vi "F2tauScale.vi"(8 "F2 channel":u8, 9 "Palette tau":T3(ring), 10 "Palette F2":T3(ring), 11 "Enum":T1(ring)) -> (0 "error out":errorcluster, 2 "tauscale":T2, 3 "F2-scale":T2, 4 "title tau":string, 5 "title F2":string)   [LabVIEW 2009]
uses:
  <vilib>/vision/Image Controls.llb/IMAQ Image.ctl
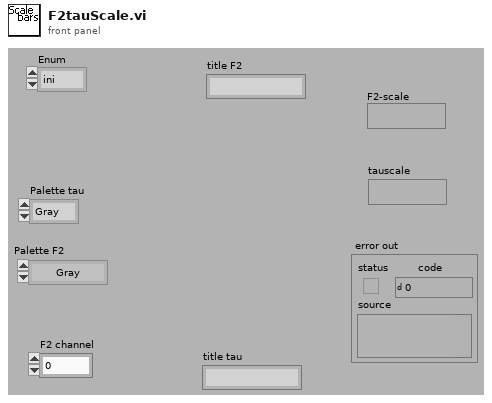
[diagram p1: front panel]
types:
  T1 = enum16{"ini", "get", "change", "export", "draw", "dump", "kill", "colorpal"}
  T2 = typedef "IMAQ Image.ctl" = refnum<image>
  T3 = enum32{"Gray", "Binary", "Gradient", "Rainbow", "Temperature"}
  T4 = typedef "Settings.ctl" = cluster{"threshold":cluster{"max":u32, "min":u32}, "RGB or false color":bool, "16bit":bool, "log/lin axis":u16, "spotsize button":bool, "Pixelsize":u16, "autoscale x":bool, "autoscale y":bool, "correlation":bool, "ADC-Resolution":i32, "F2-lifetime":cluster{"display tau":bool, "display F2":bool, "Palette Number lifetime":enum32{"Gray", "Binary", "Gradient", "Rainbow", "Temperature"}, "Palette Number F2":enum32{"Gray", "Binary", "Gradient", "Rainbow", "Temperature"}, "max tau-Value":dbl, "min tau-Value":dbl, "max F2-Value":dbl, "min F2-Value":dbl}, "TAC-Window 1":u16, "TAC-Window 2":u16, "false color palette":cluster{"1":u32, "2":u32, "3":u32, "4":u32, "5":u32, "6":u32, "7":u32, "8":u32, "8 2":u32, "8 3":u32, "8 4":u32, "8 5":u32}}
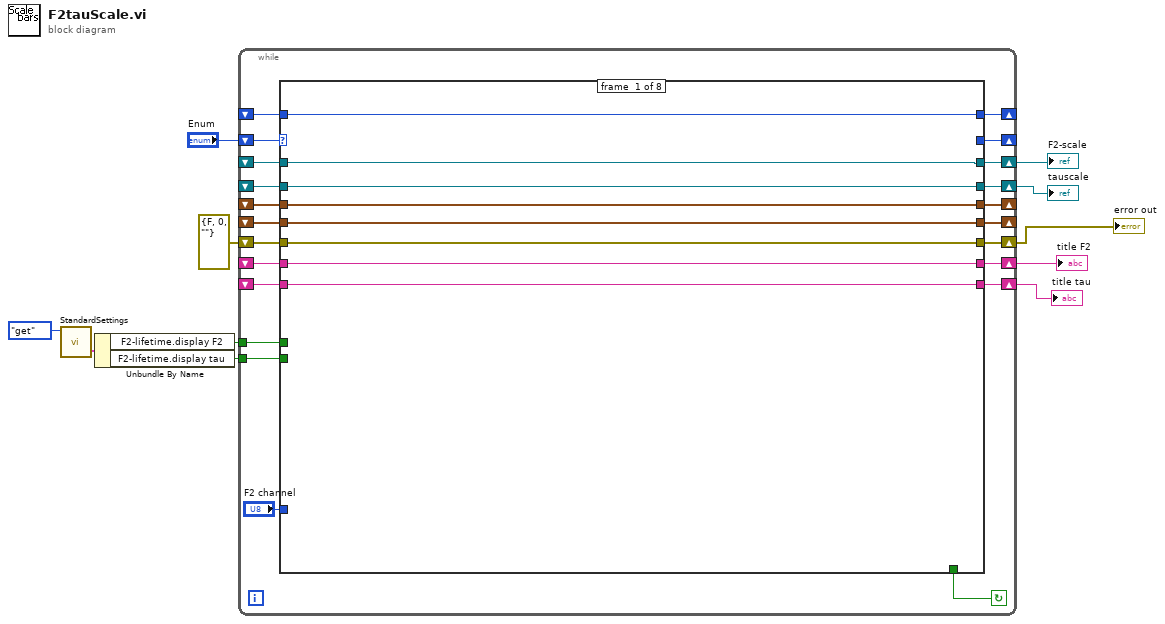
[diagram p0: block diagram]
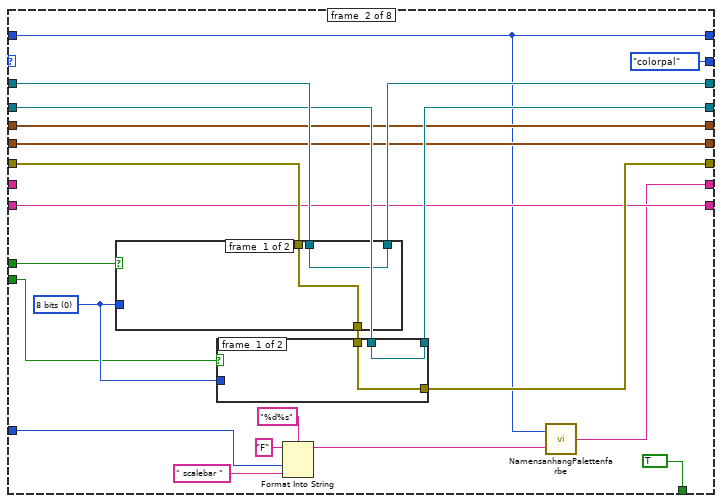
[diagram p2: hidden frame]
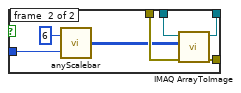
[diagram p3: hidden frame]
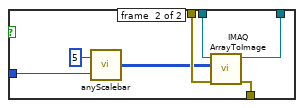
[diagram p4: hidden frame]
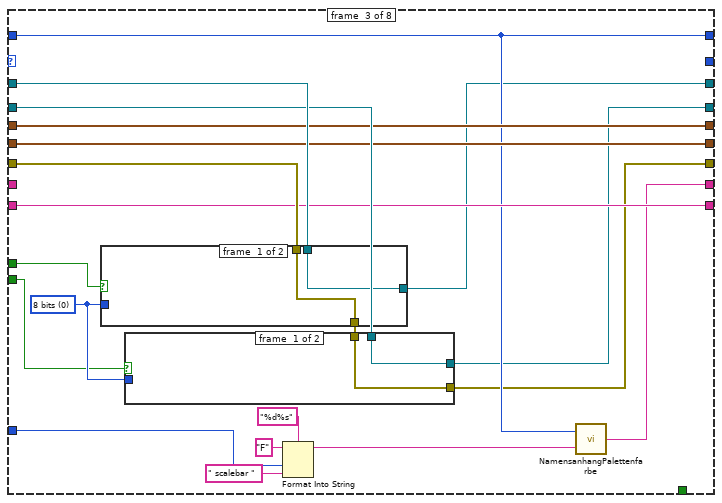
[diagram p5: hidden frame]
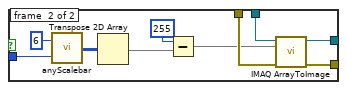
[diagram p6: hidden frame]
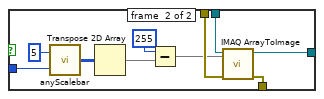
[diagram p7: hidden frame]
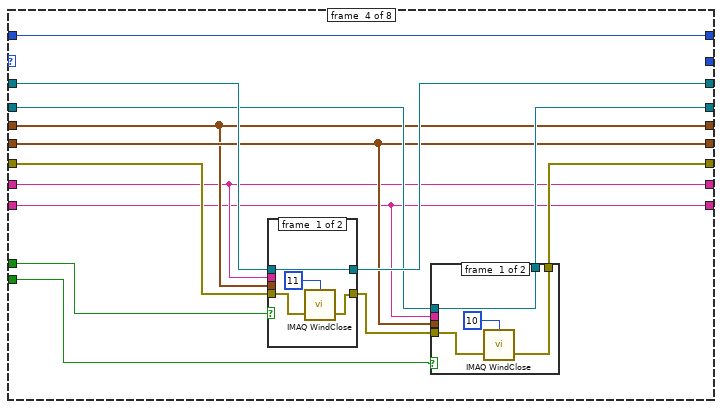
[diagram p8: hidden frame]
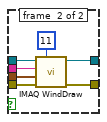
[diagram p9: hidden frame]
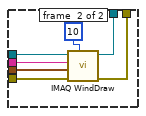
[diagram p10: hidden frame]
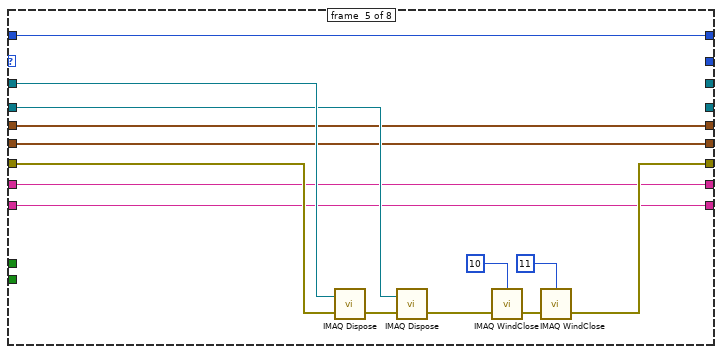
[diagram p11: hidden frame]
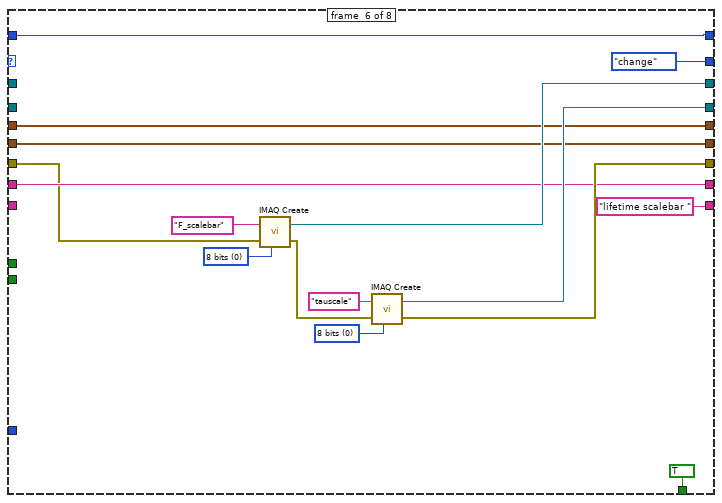
[diagram p12: hidden frame]
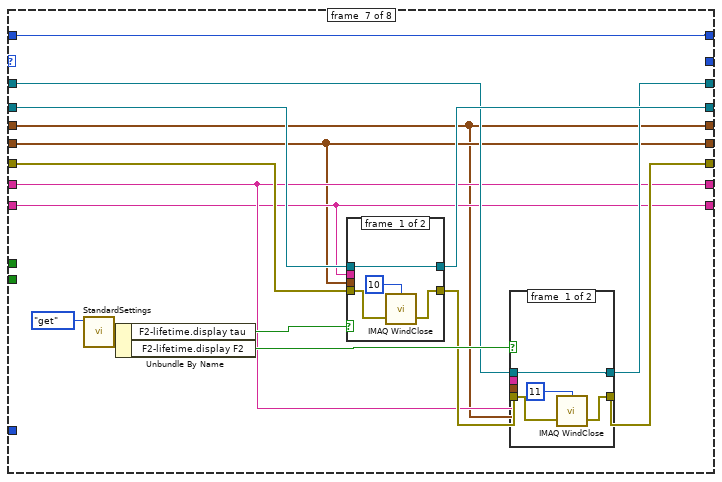
[diagram p13: hidden frame]
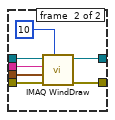
[diagram p14: hidden frame]
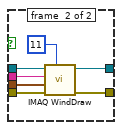
[diagram p15: hidden frame]
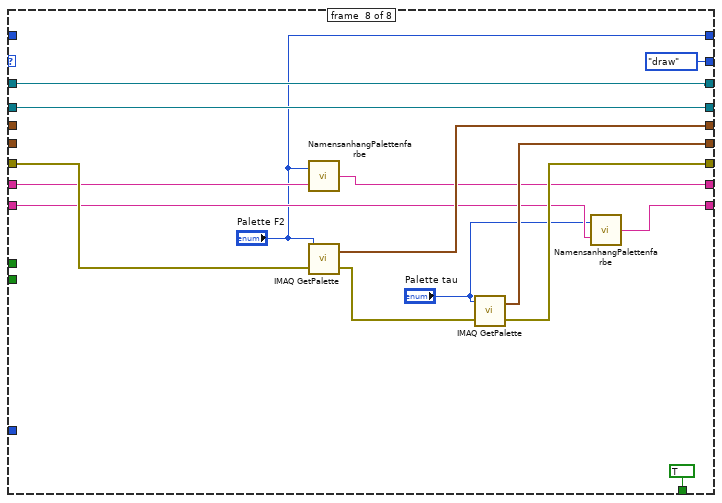
[diagram p16: hidden frame]
diagram:
  n1 = call "StandardSettings.vi"("Enum"=enum16{"Load", "get", "Save", "set"}."get") -> ("StandardSettings"=w3:T4)  [unwired: 4 in]
  n2 = Unbundle By Name(w3) -> ("F2-lifetime.display F2"=w2:bool, "F2-lifetime.display tau"=w1:bool)
  n3 = while {
    shift-right: [w32] -> _
    shift-left: "Enum" -> [w33]
    shift-right: [w31] -> w10
    shift-left: _ -> [w28]
    shift-right: [w30] -> w9
    shift-left: _ -> [w27]
    shift-right: [w24] -> _
    shift-left: _ -> [w22]
    shift-right: [w29] -> w5
    shift-left: errorcluster {"status"=FALSE, "code"=0, "source"=""} ("error out") -> [w26]
    shift-right: [w23] -> _
    shift-left: _ -> [w21]
    shift-right: [w20] -> w7
    shift-left: _ -> [w19]
    shift-right: [w16] -> w6
    shift-left: _ -> [w17]
    shift-right: [w15] -> _
    shift-left: _ -> [w14]
    tunnel: w2 -> [w13]
    tunnel: w1 -> [w12]
    stop <- w25 continue-if-true
    n4 = case shown="\"draw\"" w33 {
      tunnel: [_ T1."colorpal" ("Enum") _ _ _ T1."change" ("Enum") _ T1."draw" ("Enum")] -> w32
      tunnel: [w41 w56 w86 w138 _ w186 w200 w239] -> w31
      tunnel: [w40 w57 w84 w135 _ w185 w202 w238] -> w30
      tunnel: [w39 w59 w85 w131 w169 w184 w197 w241] -> w29
      tunnel: w28 -> [w41 w62 w100 w137 w175 _ w201 w239]
      tunnel: w27 -> [w40 w58 w97 w136 w174 _ w203 w238]
      tunnel: w26 -> [w39 w61 w99 w132 w172 w180 w199 w240]
      tunnel: [_ TRUE _ _ _ TRUE _ TRUE] -> w25
      tunnel: [w38 w54 w96 w133 w166 w183 w192 w244] -> w24
      tunnel: [w37 w53 w95 w134 w165 w182 w193 w243] -> w23
      tunnel: w22 -> [w38 w54 w96 w133 w166 w183 w192 _]
      tunnel: w21 -> [w37 w53 w95 w134 w165 w182 w193 _]
      tunnel: [w36 w45 w87 w130 w164 w181 w196 w236] -> w20
      tunnel: w19 -> [w36 _ _ w130 w164 w181 w196 w237]
      tunnel: "F2 channel" -> [_ w49 w91 _ _ _ _ _]
      tunnel: w17 -> [w35 w48 w90 w129 w163 _ w195 w235]
      tunnel: [w35 w48 w90 w129 w163 "lifetime scalebar " ("Title") w195 w233] -> w16
      tunnel: [w34 w46 w88 w128 w162 w178 w194 "Palette F2"] -> w15
      tunnel: w14 -> [w34 w46 w88 w128 w162 w178 w194 _]
      tunnel: w13 -> [_ w43 w83 w127 _ _ _ _]
      tunnel: w12 -> [_ w42 w82 w126 _ _ _ _]
      frame #0 {
      }
      frame #1 {
        w63 = u32 0 items=["8 bits", "16 bits", "Float", "Complex", "RGB", "HSL"] ("Image Type")
        n5 = case shown="False" w43 {
          tunnel: w63 -> [_ w80]
          tunnel: w62 -> [w74 w79]
          tunnel: w61 -> [w73 w78]
          tunnel: [w73 w77] -> w60
          tunnel: [w74 w76] -> w56
          frame #0 {
          }
          frame #1 {
            n6 = call "anyScalebar.vi"("Image Type"=w80, "Window Number"=5) -> ("Image Pixels (I16)"=w75:i16[][])
            n7 = call "IMAQ ArrayToImage"("error in (no error)"=w78, "Image Pixels (U8)"=w75, "Image"=w79) -> ("error out"=w77:errorcluster, "Image Out"=w76:T2)  [unwired: 7 in]
          }
        }
        n8 = case shown="True" w42 {
          tunnel: w63 -> [_ w71]
          tunnel: w60 -> [w64 w70]
          tunnel: [w64 w69] -> w59
          tunnel: w58 -> [w65 w68]
          tunnel: [w65 w67] -> w57
          frame #0 {
          }
          frame #1 {
            n9 = call "anyScalebar.vi"("Image Type"=w71, "Window Number"=6) -> ("Image Pixels (I16)"=w66:i16[][])
            n10 = call "IMAQ ArrayToImage"("error in (no error)"=w70, "Image Pixels (U8)"=w66, "Image"=w68) -> ("error out"=w69:errorcluster, "Image Out"=w67:T2)  [unwired: 7 in]
          }
        }
        n11 = Format Into String(format string="%d%s", initial string="F", w49, " scalebar " ("input 3")) -> (resulting string=w47:string)  [unwired: 1 in, 1 out]
        n12 = call "NamensanhangPalettenfarbe.vi"("String"=w47, "Palette F2"=w46) -> ("String"=w45:string)
      }
      frame #2 {
        w101 = u32 0 items=["8 bits", "16 bits", "Float", "Complex", "RGB", "HSL"] ("Image Type")
        n13 = case shown="True" w83 {
          tunnel: w101 -> [_ w124]
          tunnel: w100 -> [w114 w123]
          tunnel: w99 -> [w115 w122]
          tunnel: [w115 w121] -> w98
          tunnel: [w114 w120] -> w86
          frame #0 {
          }
          frame #1 {
            n14 = call "anyScalebar.vi"("Image Type"=w124, "Window Number"=5) -> ("Image Pixels (I16)"=w119:i16[][])
            n15 = Transpose 2D Array(2D array=w119) -> (transposed array=w118:i16[][])
            n16 = Subtract(x=i16 255, y=w118) -> (x-y=w116:i16[][])
            n17 = call "IMAQ ArrayToImage"("error in (no error)"=w122, "Image Pixels (U8)"=w116, "Image"=w123) -> ("error out"=w121:errorcluster, "Image Out"=w120:T2)  [unwired: 7 in]
          }
        }
        n18 = case shown="True" w82 {
          tunnel: w101 -> [_ w112]
          tunnel: w98 -> [w103 w111]
          tunnel: w97 -> [w102 w110]
          tunnel: [w103 w109] -> w85
          tunnel: [w102 w108] -> w84
          frame #0 {
          }
          frame #1 {
            n19 = call "anyScalebar.vi"("Image Type"=w112, "Window Number"=6) -> ("Image Pixels (I16)"=w107:i16[][])
            n20 = Transpose 2D Array(2D array=w107) -> (transposed array=w105:i16[][])
            n21 = Subtract(x=i16 255, y=w105) -> (x-y=w104:i16[][])
            n22 = call "IMAQ ArrayToImage"("error in (no error)"=w111, "Image Pixels (U8)"=w104, "Image"=w110) -> ("error out"=w109:errorcluster, "Image Out"=w108:T2)  [unwired: 7 in]
          }
        }
        n23 = Format Into String(format string="%d%s", initial string="F", w91, " scalebar " ("input 3")) -> (resulting string=w89:string)  [unwired: 1 in, 1 out]
        n24 = call "NamensanhangPalettenfarbe.vi"("String"=w89, "Palette F2"=w88) -> ("String"=w87:string)
      }
      frame #3 {
        n25 = case shown="False" w127 {
          tunnel: [w140 w149] -> w139
          tunnel: [w143 w148] -> w138
          tunnel: w137 -> [w143 w147]
          tunnel: w133 -> [_ w146]
          tunnel: w132 -> [w141 w145]
          tunnel: w130 -> [_ w144]
          frame #0 {
            n26 = call "IMAQ WindClose"("Window Number (0...15)"=11, "error in (no error)"=w141) -> ("error out"=w140:errorcluster)  [unwired: 4 in]
          }
          frame #1 {
            n27 = call "IMAQ WindDraw"("Window Number (0...15)"=11, "error in (no error)"=w145, "Color Palette"=w146, "Title"=w144, "Image"=w147) -> ("error out"=w149:errorcluster, "Image Out (duplicate)"=w148:T2)  [unwired: 5 in]
          }
        }
        n28 = case shown="True" w126 {
          tunnel: w139 -> [w152 w160]
          tunnel: w136 -> [w154 w159]
          tunnel: [w154 w158] -> w135
          tunnel: w134 -> [_ w157]
          tunnel: [w151 w156] -> w131
          tunnel: w129 -> [_ w155]
          frame #0 {
            n29 = call "IMAQ WindClose"("Window Number (0...15)"=10, "error in (no error)"=w152) -> ("error out"=w151:errorcluster)  [unwired: 4 in]
          }
          frame #1 {
            n30 = call "IMAQ WindDraw"("Window Number (0...15)"=10, "error in (no error)"=w160, "Color Palette"=w157, "Title"=w155, "Image"=w159) -> ("error out"=w156:errorcluster, "Image Out (duplicate)"=w158:T2)  [unwired: 5 in]
          }
        }
      }
      frame #4 {
        n31 = call "IMAQ Dispose"("Image"=w175, "error in (no error)"=w172) -> ("error out"=w173:errorcluster)  [unwired: 4 in]
        n32 = call "IMAQ Dispose"("Image"=w174, "error in (no error)"=w173) -> ("error out"=w171:errorcluster)  [unwired: 4 in]
        n33 = call "IMAQ WindClose"("Window Number (0...15)"=10, "error in (no error)"=w171) -> ("error out"=w170:errorcluster)  [unwired: 4 in]
        n34 = call "IMAQ WindClose"("Window Number (0...15)"=11, "error in (no error)"=w170) -> ("error out"=w169:errorcluster)  [unwired: 4 in]
      }
      frame #5 {
        w187 = u32 0 items=["8 bits", "16 bits", "Float", "Complex", "RGB", "HSL"] ("Image Type")
        w188 = u32 0 items=["8 bits", "16 bits", "Float", "Complex", "RGB", "HSL"] ("Image Type")
        n35 = call "IMAQ Create"("Image Name"="F_scalebar", "Image Type"=w187, "error in (no error)"=w180) -> ("New Image"=w186:T2, "error out"=w190:errorcluster)  [unwired: 2 in]
        n36 = call "IMAQ Create"("Image Name"="tauscale", "Image Type"=w188, "error in (no error)"=w190) -> ("New Image"=w185:T2, "error out"=w184:errorcluster)  [unwired: 2 in]
      }
      frame #6 {
        n37 = call "StandardSettings.vi"("Enum"=enum16{"Load", "get", "Save", "set"}."get") -> ("StandardSettings"=w207:T4)  [unwired: 4 in]
        n38 = Unbundle By Name(w207) -> ("F2-lifetime.display tau"=w205:bool, "F2-lifetime.display F2"=w204:bool)
        n39 = case shown="False" w205 {
          tunnel: w203 -> [w210 w217]
          tunnel: [w210 w216] -> w202
          tunnel: w193 -> [_ w215]
          tunnel: w199 -> [w209 w214]
          tunnel: [w208 w213] -> w198
          tunnel: w195 -> [_ w212]
          frame #0 {
            n40 = call "IMAQ WindClose"("Window Number (0...15)"=10, "error in (no error)"=w209) -> ("error out"=w208:errorcluster)  [unwired: 4 in]
          }
          frame #1 {
            n41 = call "IMAQ WindDraw"("Window Number (0...15)"=10, "error in (no error)"=w214, "Color Palette"=w215, "Title"=w212, "Image"=w217) -> ("error out"=w213:errorcluster, "Image Out (duplicate)"=w216:T2)  [unwired: 5 in]
          }
        }
        n42 = case shown="False" w204 {
          tunnel: w201 -> [w221 w228]
          tunnel: [w221 w227] -> w200
          tunnel: w192 -> [_ w226]
          tunnel: w198 -> [w220 w225]
          tunnel: [w219 w224] -> w197
          tunnel: w196 -> [_ w223]
          frame #0 {
            n43 = call "IMAQ WindClose"("Window Number (0...15)"=11, "error in (no error)"=w220) -> ("error out"=w219:errorcluster)  [unwired: 4 in]
          }
          frame #1 {
            n44 = call "IMAQ WindDraw"("Window Number (0...15)"=11, "error in (no error)"=w225, "Color Palette"=w226, "Title"=w223, "Image"=w228) -> ("error out"=w224:errorcluster, "Image Out (duplicate)"=w227:T2)  [unwired: 5 in]
          }
        }
      }
      frame #7 {
        n45 = call "NamensanhangPalettenfarbe.vi"("String"=w237, "Palette F2"="Palette F2") -> ("String"=w236:string)
        n46 = call "IMAQ GetPalette"("Palette Number (gray)"="Palette F2", "error in (no error)"=w240) -> ("Color Palette"=w244:cluster{"Red":u8, "Green":u8, "Blue":u8}[], "error out"=w242:errorcluster)  [unwired: 3 in]
        n47 = call "IMAQ GetPalette"("Palette Number (gray)"="Palette tau", "error in (no error)"=w242) -> ("Color Palette"=w243:cluster{"Red":u8, "Green":u8, "Blue":u8}[], "error out"=w241:errorcluster)  [unwired: 3 in]
        n48 = call "NamensanhangPalettenfarbe.vi"("String"=w235, "Palette F2"="Palette tau") -> ("String"=w233:string)
      }
    }
  }
  "error out" <- w5
  "tauscale" <- w9
  "F2-scale" <- w10
  "title F2" <- w7
  "title tau" <- w6
